vi "Update_Menu_Items.vi"(6 "Menu Type":enum16{"Root", "Sub", "Child"}(ring), 7 "Menu":refnum<vi>, 8 "error in":errorcluster, 10 "Parent Menu Name":string, 11 "Menu_Configuration":T1={"Button_Label_Color"=2344, "Button_Color_On"=5654, "Button_Color_Off"=2344, "Panel_Color"=2344, "Extend_Sub_Menu_Icon"=path "C:/Users/SyncSols-4/Desktop/Icon/Accept-icon.png", "Root_Menu_Data"=[{"Button_Icon"=path "C:/Users/SyncSols-4/Desktop/Icon/Accept-icon.png", "Button_Label"="Test", "Sub_Menu_Data"=[{"Button_Icon"=path "C:/Users/SyncSols-4/Desktop/Icon/floppy-icon.png", "Button_Label"="Save", "Child_Menu_Data"=[]}, {"Button_Icon"=path "C:/Users/SyncSols-4/Desktop/Icon/folder-icon1.png", "Button_Label"="Folder", "Child_Menu_Data"=[]}, {"Button_Icon"=path "C:/Users/SyncSols-4/Desktop/Icon/delete-icon.png", "Button_Label"="Delete", "Child_Menu_Data"=[{"Button_Icon"=path "C:/Users/SyncSols-4/Desktop/Icon/add-icon.png", "Button_Label"="Add"}, {"Button_Icon"=path "C:/Users/SyncSols-4/Desktop/Icon/Stop-red-icon.png", "Button_Label"="Stop"}]}]}, {"Button_Icon"=path "C:/Users/SyncSols-4/Desktop/Icon/add-key-icon.png", "Button_Label"="Key", "Sub_Menu_Data"=[]}, {"Button_Icon"=path "C:/Users/SyncSols-4/Desktop/Icon/Categories-preferences-system-icon.png", "Button_Label"="Setting", "Sub_Menu_Data"=[]}]}) -> (0 "error out":errorcluster)   [LabVIEW 2019]
doc: "All Rights Reserved © 2017 SyncSols"
uses:
  Controls/Menu_Configuration.ctl
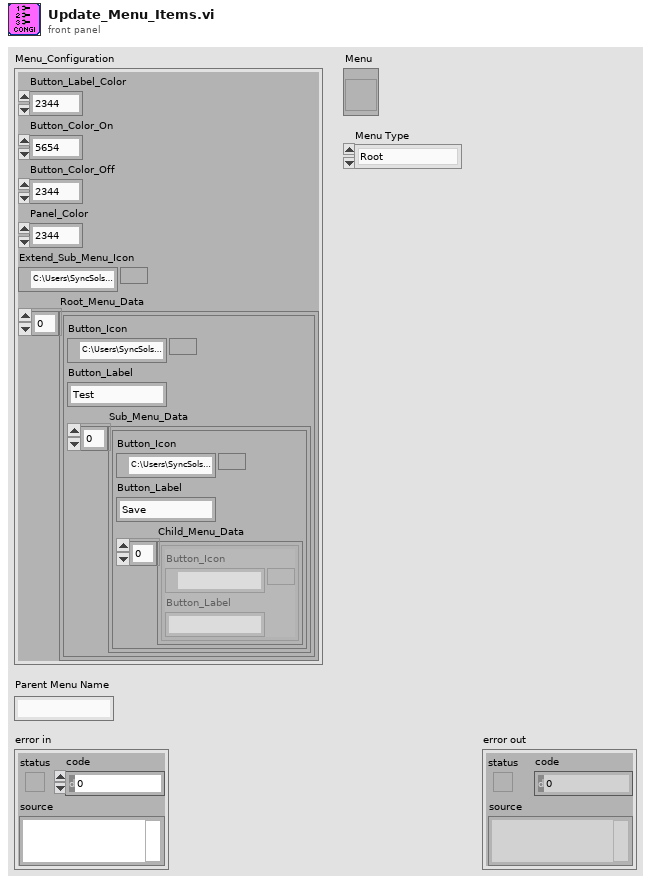
[diagram p1: front panel]
types:
  T1 = typedef "Menu_Configuration.ctl" = cluster{"Button_Label_Color":u32, "Button_Color_On":u32, "Button_Color_Off":u32, "Panel_Color":u32, "Extend_Sub_Menu_Icon":path, "Root_Menu_Data":cluster{"Button_Icon":path, "Button_Label":string, "Sub_Menu_Data":cluster{"Button_Icon":path, "Button_Label":string, "Child_Menu_Data":cluster{"Button_Icon":path, "Button_Label":string}[]}[]}[]}
  T2 = cluster{"Text ":string, "Icon":picture, "Button":bool, "Sub Menu":picture}
  T3 = cluster{"Button_Icon":path, "Button_Label":string, "Sub_Menu_Data":cluster{"Button_Icon":path, "Button_Label":string, "Child_Menu_Data":cluster{"Button_Icon":path, "Button_Label":string}[]}[]}[]
  T4 = typedef "imagedata.ctl" = cluster{"image type":i32, "image depth":i32, "image":u8[], "mask":u8[], "colors":u32[], "Rectangle":cluster{"left":i16, "top":i16, "right":i16, "bottom":i16}}
  T5 = cluster{"Button_Icon":path, "Button_Label":string, "Child_Menu_Data":cluster{"Button_Icon":path, "Button_Label":string}[]}[]
  T6 = cluster{"Button_Icon":path, "Button_Label":string}[]
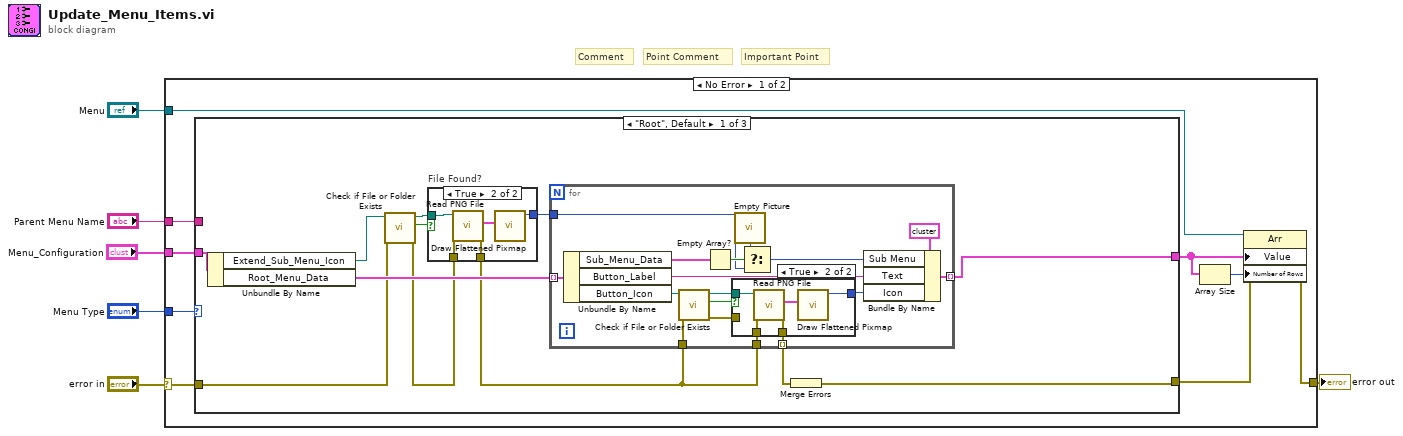
[diagram p0: block diagram]
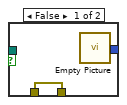
[diagram p2: hidden frame]
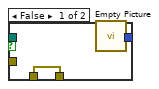
[diagram p3: hidden frame]
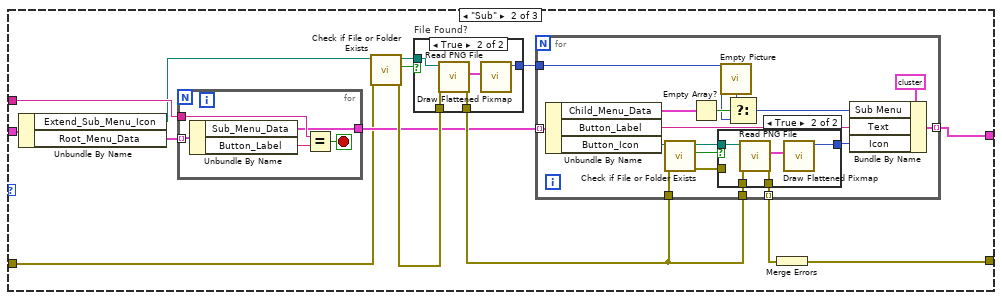
[diagram p4: hidden frame]
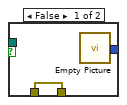
[diagram p5: hidden frame]
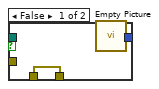
[diagram p6: hidden frame]
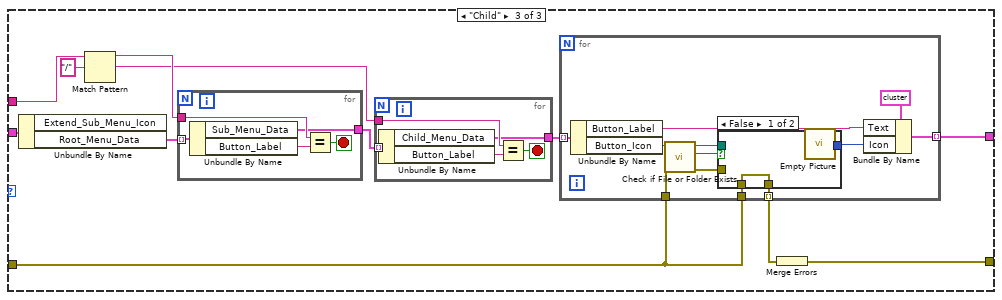
[diagram p7: hidden frame]
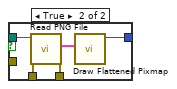
[diagram p8: hidden frame]
diagram:
  # "Important Point"
  # "Point Comment"
  # "Comment"
  n1 = case shown="No Error" "error in" {
    selector: "error in" -> [w14 w150]
    tunnel: [w9 w150] -> w6
    tunnel: "Menu Type" -> [w15 _]
    tunnel: "Menu_Configuration" -> [w13 _]
    tunnel: "Menu" -> [w12 _]
    tunnel: "Parent Menu Name" -> [w11 _]
    frame No Error {
      n2 = case shown="\"Root\", Default" w15 {
        tunnel: w14 -> [w23 w63 w111]
        tunnel: w13 -> [w27 w72 w120]
        tunnel: w11 -> [_ w70 w117]
        tunnel: [w17 w59 w110] -> w10
        tunnel: [w18 w60 w109] -> w8
        frame "Root", Default {
          n3 = Unbundle By Name(w27) -> ("Extend_Sub_Menu_Icon"=w24:path, "Root_Menu_Data"=w26:T3)
          n4 = call <vilib>:"Check if File or Folder Exists.vi"("error in (no error)"=w23, "path"=w24) -> ("error out"=w21:errorcluster, "file or folder exists?"=w22:bool, "dup path"=w16:path)  [unwired: 7 in]
          n5 = case "File Found?" shown="True" w22 {
            tunnel: [w29 w34] -> w19
            tunnel: [w28 w32] -> w25
            tunnel: w21 -> [w29 w31]
            tunnel: w16 -> [_ w30]
            frame False {
              n6 = call "Empty Picture"() -> ("empty picture"=w28:picture)
            }
            frame True {
              n7 = call <vilib>:"Read PNG File.vi"("error in (no error)"=w31, "path to PNG file"=w30) -> ("error out"=w34:errorcluster, "image data"=w33:T4)  [unwired: 7 in, 1 out]
              n8 = call <vilib>:"Draw Flattened Pixmap.vi"("image data"=w33) -> ("new picture"=w32:picture)  [unwired: 8 in]
            }
          }
          n9 = for {
            tunnel: w26 -> [w51] mode=indexing
            tunnel: w19 -> [w50]
            tunnel: w25 -> [w46]
            tunnel: [w38] -> w18 mode=indexing
            tunnel: [w37] -> w20 mode=indexing
            tunnel: w19 -> [w36]
            n10 = Unbundle By Name(w51) -> ("Sub_Menu_Data"=w48:T5, "Button_Label"=w39:string, "Button_Icon"=w45:path)
            n11 = call <vilib>:"Check if File or Folder Exists.vi"("error in (no error)"=w36, "path"=w45) -> ("error out"=w35:errorcluster, "file or folder exists?"=w44:bool, "dup path"=w43:path)  [unwired: 7 in]
            n12 = Empty Array?(array=w48) -> (empty?=w49:bool)
            n13 = case shown="True" w44 {
              tunnel: w50 -> [w52 w58]
              tunnel: w43 -> [_ w56]
              tunnel: [w53 w55] -> w40
              tunnel: [w52 w54] -> w37
              tunnel: w35 -> [_ _]
              frame False {
                n14 = call "Empty Picture"() -> ("empty picture"=w53:picture)
              }
              frame True {
                n15 = call <vilib>:"Read PNG File.vi"("error in (no error)"=w58, "path to PNG file"=w56) -> ("error out"=w54:errorcluster, "image data"=w57:T4)  [unwired: 7 in, 1 out]
                n16 = call <vilib>:"Draw Flattened Pixmap.vi"("image data"=w57) -> ("new picture"=w55:picture)  [unwired: 8 in]
              }
            }
            n17 = call "Empty Picture"() -> ("empty picture"=w47:picture)
            n18 = Select(t=w47, s=w49, f=w46) -> (s? t:f=w41:picture)
            n19 = Bundle By Name(cluster=T2 {"Text "="", "Icon"=bytes[0], "Button"=FALSE, "Sub Menu"=bytes[0]} ("Cluster 3"), "Sub Menu"=w41, "Text"=w39, "Icon"=w40) -> (w38:T2)
          }
          n20 = Merge Errors(w20) -> (w17:errorcluster)
        }
        frame "Sub" {
          n21 = Unbundle By Name(w72) -> ("Extend_Sub_Menu_Icon"=w61:path, "Root_Menu_Data"=w71:T3)
          n22 = for {
            tunnel: w71 -> [w108] mode=indexing
            tunnel: w70 -> [w106]
            tunnel: [w104] -> w64
            stop <- w105 stop-if-true
            n23 = Unbundle By Name(w108) -> ("Sub_Menu_Data"=w104:T5, "Button_Label"=w107:string)
            n24 = Equal?(x=w106, y=w107) -> (x = y?=w105:bool)
          }
          n25 = call <vilib>:"Check if File or Folder Exists.vi"("error in (no error)"=w63, "path"=w61) -> ("error out"=w67:errorcluster, "file or folder exists?"=w68:bool, "dup path"=w62:path)  [unwired: 7 in]
          n26 = case "File Found?" shown="True" w68 {
            tunnel: [w74 w79] -> w65
            tunnel: [w73 w77] -> w69
            tunnel: w67 -> [w74 w76]
            tunnel: w62 -> [_ w75]
            frame False {
              n27 = call "Empty Picture"() -> ("empty picture"=w73:picture)
            }
            frame True {
              n28 = call <vilib>:"Read PNG File.vi"("error in (no error)"=w76, "path to PNG file"=w75) -> ("error out"=w79:errorcluster, "image data"=w78:T4)  [unwired: 7 in, 1 out]
              n29 = call <vilib>:"Draw Flattened Pixmap.vi"("image data"=w78) -> ("new picture"=w77:picture)  [unwired: 8 in]
            }
          }
          n30 = for {
            tunnel: w64 -> [w96] mode=indexing
            tunnel: w65 -> [w95]
            tunnel: w69 -> [w91]
            tunnel: [w83] -> w60 mode=indexing
            tunnel: [w82] -> w66 mode=indexing
            tunnel: w65 -> [w81]
            n31 = Unbundle By Name(w96) -> ("Child_Menu_Data"=w93:T6, "Button_Label"=w84:string, "Button_Icon"=w90:path)
            n32 = call <vilib>:"Check if File or Folder Exists.vi"("error in (no error)"=w81, "path"=w90) -> ("error out"=w80:errorcluster, "file or folder exists?"=w89:bool, "dup path"=w88:path)  [unwired: 7 in]
            n33 = Empty Array?(array=w93) -> (empty?=w94:bool)
            n34 = case shown="True" w89 {
              tunnel: w95 -> [w97 w103]
              tunnel: w88 -> [_ w101]
              tunnel: [w98 w100] -> w85
              tunnel: [w97 w99] -> w82
              tunnel: w80 -> [_ _]
              frame False {
                n35 = call "Empty Picture"() -> ("empty picture"=w98:picture)
              }
              frame True {
                n36 = call <vilib>:"Read PNG File.vi"("error in (no error)"=w103, "path to PNG file"=w101) -> ("error out"=w99:errorcluster, "image data"=w102:T4)  [unwired: 7 in, 1 out]
                n37 = call <vilib>:"Draw Flattened Pixmap.vi"("image data"=w102) -> ("new picture"=w100:picture)  [unwired: 8 in]
              }
            }
            n38 = call "Empty Picture"() -> ("empty picture"=w92:picture)
            n39 = Select(t=w92, s=w94, f=w91) -> (s? t:f=w86:picture)
            n40 = Bundle By Name(cluster=T2 {"Text "="", "Icon"=bytes[0], "Button"=FALSE, "Sub Menu"=bytes[0]} ("Cluster 3"), "Sub Menu"=w86, "Text"=w84, "Icon"=w85) -> (w83:T2)
          }
          n41 = Merge Errors(w66) -> (w59:errorcluster)
        }
        frame "Child" {
          n42 = Unbundle By Name(w120) -> ("Root_Menu_Data"=w119:T3)  [unwired: 1 out]
          n43 = Match Pattern(string=w117, regular expression="/") -> (before substring=w115:string, after substring=w113:string)  [unwired: 1 in, 2 out]
          n44 = for {
            tunnel: w119 -> [w149] mode=indexing
            tunnel: w115 -> [w147]
            tunnel: [w145] -> w114
            stop <- w146 stop-if-true
            n45 = Unbundle By Name(w149) -> ("Sub_Menu_Data"=w145:T5, "Button_Label"=w148:string)
            n46 = Equal?(x=w147, y=w148) -> (x = y?=w146:bool)
          }
          n47 = for {
            tunnel: w114 -> [w125] mode=indexing
            tunnel: w113 -> [w123]
            tunnel: [w121] -> w112
            stop <- w122 stop-if-true
            n48 = Unbundle By Name(w125) -> ("Child_Menu_Data"=w121:T6, "Button_Label"=w124:string)
            n49 = Equal?(x=w123, y=w124) -> (x = y?=w122:bool)
          }
          n50 = for {
            tunnel: w112 -> [w137] mode=indexing
            tunnel: [w130] -> w109 mode=indexing
            tunnel: [w129] -> w118 mode=indexing
            tunnel: w111 -> [w127]
            tunnel: w111 -> [w126]
            n51 = Unbundle By Name(w137) -> ("Button_Label"=w131:string, "Button_Icon"=w136:path)
            n52 = call <vilib>:"Check if File or Folder Exists.vi"("error in (no error)"=w127, "path"=w136) -> ("error out"=w128:errorcluster, "file or folder exists?"=w135:bool, "dup path"=w134:path)  [unwired: 7 in]
            n53 = case shown="False" w135 {
              tunnel: w134 -> [_ w143]
              tunnel: [w139 w142] -> w132
              tunnel: [w138 w141] -> w129
              tunnel: w128 -> [_ _]
              tunnel: w126 -> [w138 w140]
              frame False {
                n54 = call "Empty Picture"() -> ("empty picture"=w139:picture)
              }
              frame True {
                n55 = call <vilib>:"Read PNG File.vi"("error in (no error)"=w140, "path to PNG file"=w143) -> ("error out"=w141:errorcluster, "image data"=w144:T4)  [unwired: 7 in, 1 out]
                n56 = call <vilib>:"Draw Flattened Pixmap.vi"("image data"=w144) -> ("new picture"=w142:picture)  [unwired: 8 in]
              }
            }
            n57 = Bundle By Name(cluster=T2 {"Text "="", "Icon"=bytes[0], "Button"=FALSE, "Sub Menu"=bytes[0]} ("Cluster 3"), "Text"=w131, "Icon"=w132) -> (w130:T2)
          }
          n58 = Merge Errors(w118) -> (w110:errorcluster)
        }
      }
      n59 = Array Size(array=w8) -> (size(s)=w7:i32)
      n60 = property class="Arr"(reference=w12, error in=w10, "Value"=w8, "Number of Rows"=w7) -> (error out=w9:errorcluster)  [unwired: 1 out]
    }
    frame Error {
    }
  }
  "error out" <- w6
